vi "Script FGV.vi"(11 "Action":T1) -> (2 "Button":T2)   [LabVIEW 2016]
uses:
  Controls/Action Button.ctl
  Controls/FGV Action.ctl
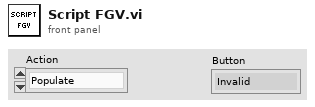
[diagram p1: front panel]
types:
  T1 = typedef "FGV Action.ctl" = enum16{"Populate", "Run", "Pause", "Stop"}
  T2 = typedef "Action Button.ctl" = enum16{"Invalid", "Start", "Execute", "Transition"}
  T3 = enum16{"Invalid", "Start", "Execute", "Transition"}
  T4 = cluster{"Button":enum16{"Invalid", "Start", "Execute", "Transition"}, "Duration":dbl}[]
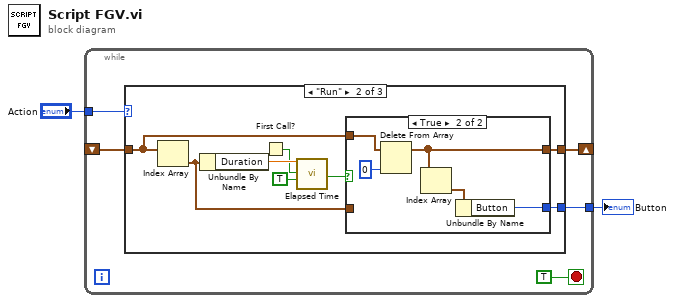
[diagram p0: block diagram]
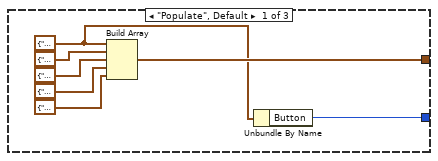
[diagram p2: hidden frame]
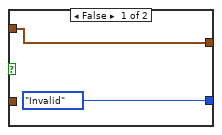
[diagram p3: hidden frame]
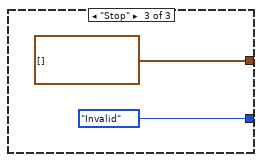
[diagram p4: hidden frame]
diagram:
  n1 = while {
    tunnel: "Action" -> [w7]
    shift-right: [w6] -> _
    shift-left: _ -> [w5]
    tunnel: [w4] -> w1
    stop <- TRUE stop-if-true
    n2 = case shown="\"Run\"" w7 {
      tunnel: [w10 w18 T4 []] -> w6
      tunnel: w5 -> [_ w20 _]
      tunnel: [w8 w16 T3."Invalid" ("Button")] -> w4
      frame "Populate", Default {
        w9 = cluster{"Button":T2, "Duration":dbl} {"Button"=enum."Start", "Duration"=10.0}
        n3 = Build Array(w9, cluster{"Button":T2, "Duration":dbl} {"Button"=enum."Execute", "Duration"=120.0}, cluster{"Button":T2, "Duration":dbl} {"Button"=enum."Transition", "Duration"=120.0}, cluster{"Button":T2, "Duration":dbl} {"Button"=enum."Transition", "Duration"=180.0}, cluster{"Button":T2, "Duration":dbl} {"Button"=enum."Execute", "Duration"=180.0}) -> (w10:cluster{"Button":T2, "Duration":dbl}[])
        n4 = Unbundle By Name(w9) -> ("Button"=w8:T2)
      }
      frame "Run" {
        n5 = Index Array(array=w20) -> (element=w17:cluster{"Button":T2, "Duration":dbl})  [unwired: 1 in]
        n6 = Unbundle By Name(w17) -> ("Duration"=w22:dbl)
        n7 = First Call?() -> (First Call?: T/F=w15:bool)
        n8 = call "Elapsed Time"("Time Target (s)"=w22, "Reset"=w15, "Auto Reset"=TRUE) -> ("Time has Elapsed"=w19:bool)  [unwired: 9 in, 7 out]
        n9 = case shown="True" w19 {
          tunnel: w20 -> [w23 w29]
          tunnel: [w23 w26] -> w18
          tunnel: w17 -> [_ _]
          tunnel: [T3."Invalid" ("Button") w27] -> w16
          frame False {
          }
          frame True {
            n10 = Delete From Array(array=w29, index=0) -> (array with subset deleted=w26:cluster{"Button":T2, "Duration":dbl}[])  [unwired: 1 in, 1 out]
            n11 = Index Array(array=w26) -> (element=w25:cluster{"Button":T2, "Duration":dbl})  [unwired: 1 in]
            n12 = Unbundle By Name(w25) -> ("Button"=w27:T2)
          }
        }
      }
      frame "Stop" {
      }
    }
  }
  "Button" <- w1
